vi "Agilent ENA Series Configuration Application.vi"() -> ()   [LabVIEW 2022 SP3]
doc: "Configures instrument for measurement."
uses:
  <instrlib>/Agilent Ena Series/Agilent ENA Series.lvlib
panel:
  in  "Reset? (T: Yes)":bool=TRUE
  in  "ID Query? (T: Yes)":bool=TRUE
  in  "Power Level (0.0)":dbl=-10.0 format="%^.2g"
  in  "IF Bandwidth":dbl=10000.0 format="%^.2e"
  in  "Span Frequency [Hz]":dbl=200000000.0 format="%^.2e"
  in  "Center Frequency [Hz]":dbl=947500000.0 format="%^.2e"
  in  "VISA resource name":refnum<visa-resource-name>
  # "(c) 2005-2021 National Instruments.  ALL RIGHTS RESERVED."
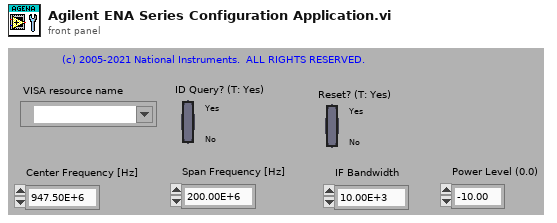
[diagram p1: front panel]
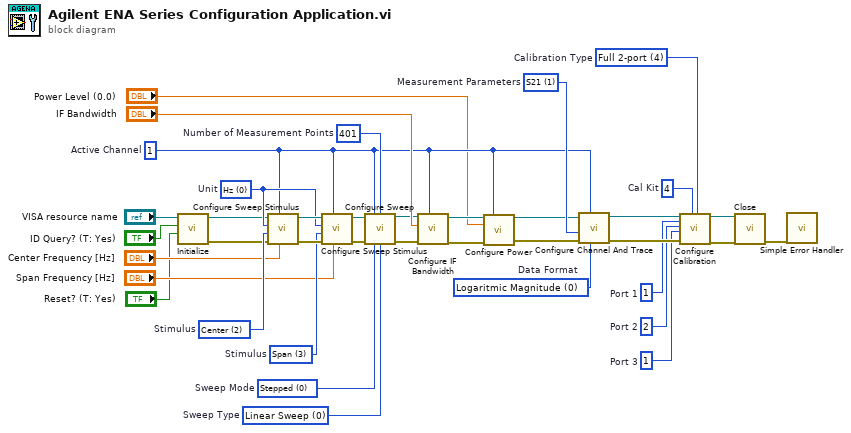
[diagram p0: block diagram]
diagram:
  w5 = u16 0 items=["Logaritmic Magnitude", "Phase", "Group Delay", "Smith Chart  Linear (Lin/Phase)", "Smith Chart  Logaritmic (Log/Phase)", "Smith Chart  Complex (Real/Imag)", "Smith Chart  Impedance (R+jX)", "Smith Chart  Admittance (G+jB)", "Polar Format (Linear)", "Polar Format (Logaritmic)", "Polar Format (Re/Im)", "Linear Magnitude", "SWR", "Real", "Imaginary", "Epanded Phase", "Positive Phase"]  # Data Format
  w6 = 4  # Cal Kit
  w7 = 2  # Port 2
  w8 = 1  # Port 3
  w9 = 1  # Port 1
  w10 = u16 4 items=["Open", "Short", "Through", "1-port", "Full 2-port", "Full 3-port", "Full 4-port"]  # Calibration Type
  w26 = u16 0 items=["Linear Sweep", "Logaritmic Sweep", "Segment Sweep", "Power Sweep"]  # Sweep Type
  w27 = 401  # Number of Measurement Points
  w28 = u16 0 items=["Stepped", "Swept", "Fast Stepped Mode", "Fast Swept Mode"]  # Sweep Mode
  w31 = u16 3 items=["Start", "Stop", "Center", "Span"]  # Stimulus
  w29 = u16 0 items=["Hz", "kHz", "MHz", "GHz", "dBm", "s"]  # Unit
  w35 = u16 2 items=["Start", "Stop", "Center", "Span"]  # Stimulus
  w36 = u16 1 items=["S11", "S21", "S31", "S41", "S12", "S22", "S32", "S42", "S13", "S23", "S33", "S43", "S14", "S24", "S34", "S44", "A", "B", "C", "D", "R1", "R2", "R3", "R4"]  # Measurement Parameters
  w4 = 1  # Active Channel
  n1 = call <instrlib>:"Initialize.vi"("Reset? (T: Yes)"="Reset? (T: Yes)", "ID Query? (T: Yes)"="ID Query? (T: Yes)", "VISA resource name"="VISA resource name") -> ("error out"=w19:errorcluster, "VISA resource name out"=w20:refnum<visa-resource-name>)  [unwired: 7 in]
  n2 = call <instrlib>:"Configure Sweep Stimulus.vi"("Parameter (0.0)"="Center Frequency [Hz]", "Channel (1)"=w4, "error in (no error)"=w19, "Stimulus (0: Start)"=w35, "Unit (0: Hz)"=w29, "VISA resource name"=w20) -> ("error out"=w33:errorcluster, "VISA resource name out"=w32:refnum<visa-resource-name>)  [unwired: 4 in]
  n3 = call <instrlib>:"Configure Sweep Stimulus.vi"("Parameter (0.0)"="Span Frequency [Hz]", "Channel (1)"=w4, "error in (no error)"=w33, "Stimulus (0: Start)"=w31, "Unit (0: Hz)"=w29, "VISA resource name"=w32) -> ("error out"=w25:errorcluster, "VISA resource name out"=w24:refnum<visa-resource-name>)  [unwired: 4 in]
  n4 = call <instrlib>:"Configure Sweep.vi"("VISA resource name"=w24, "Channel (1)"=w4, "Number of Measurement Points (201)"=w27, "error in (no error)"=w25, "Sweep Mode (0: Stepped)"=w28, "Sweep Type (0: Linear Sweep)"=w26) -> ("VISA resource name out"=w22:refnum<visa-resource-name>, "error out"=w21:errorcluster)  [unwired: 8 in]
  n5 = call <instrlib>:"Configure IF Bandwidth.vi"("Channel (1)"=w4, "error in (no error)"=w21, "IF Bandwidth (100000.0)"="IF Bandwidth", "VISA resource name"=w22) -> ("error out"=w18:errorcluster, "VISA resource name out"=w17:refnum<visa-resource-name>)  [unwired: 6 in]
  n6 = call <instrlib>:"Configure Power.vi"("VISA resource name"=w17, "Channel (1)"=w4, "Power Level (0.0)"="Power Level (0.0)", "error in (no error)"=w18) -> ("VISA resource name out"=w16:refnum<visa-resource-name>, "error out"=w15:errorcluster)  [unwired: 10 in]
  n7 = call <instrlib>:"Configure Channel And Trace.vi"("Data Format (0: Logarithmic Magnitude)"=w5, "Active Channel (1)"=w4, "error in (no error)"=w15, "Measurement Parameters (0: S11)"=w36, "VISA resource name"=w16) -> ("error out"=w14:errorcluster, "VISA resource name out"=w13:refnum<visa-resource-name>)  [unwired: 5 in]
  n8 = call <instrlib>:"Configure Calibration.vi"("VISA resource name"=w13, "Port 1 (1)"=w9, "Port 2 (1)"=w7, "Port 3 (1)"=w8, "error in (no error)"=w14, "Cal Kit (1)"=w6, "Calibration Type (6: Full 4-port)"=w10) -> ("VISA resource name out"=w11:refnum<visa-resource-name>, "error out"=w12:errorcluster)  [unwired: 11 in]
  n9 = call <instrlib>:"Close.vi"("error in (no error)"=w12, "VISA resource name"=w11) -> ("error out"=w38:errorcluster)  [unwired: 9 in]
  n10 = call <vilib>:"Simple Error Handler.vi"("error in (no error)"=w38) -> ()  [unwired: 4 in, 5 out]
